vi "Image To From U32[].vi"(9 "U32[]":u32[](array[numeric]), 10 "Img In":T1) -> (1 "U32[] out":u32[](array[numeric]), 2 "Img":T1)   [LabVIEW 2021]
uses:
  <vilib>/picture/picture.llb/imagedata.ctl
  <vilib>/Utility/Data Type/NI_Data Type.lvlib
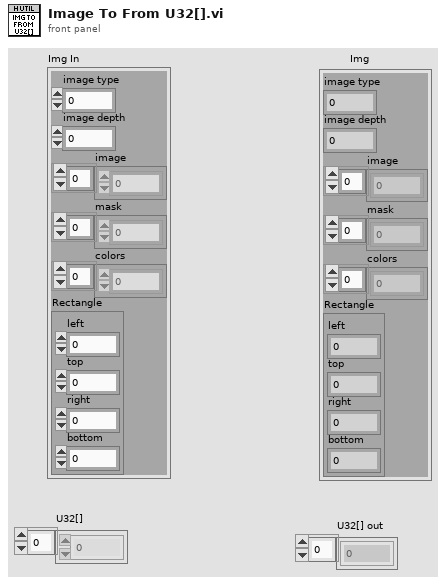
[diagram p1: front panel]
types:
  T1 = typedef "imagedata.ctl" = cluster{"image type":i32, "image depth":i32, "image":u8[], "mask":u8[], "colors":u32[], "Rectangle":cluster{"left":i16, "top":i16, "right":i16, "bottom":i16}}
  T2 = enum16{"Type", "Depth", "Sz & Image", "Sz & Mask", "Sz & Colors", "Rect"}
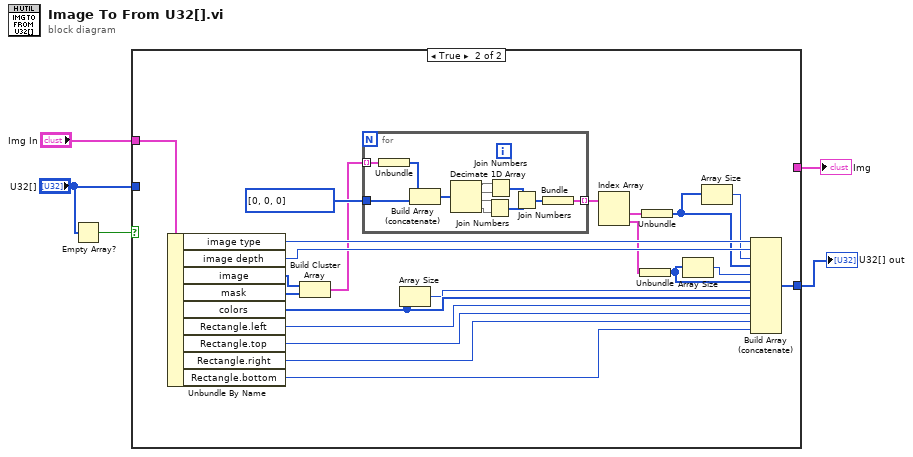
[diagram p0: block diagram]
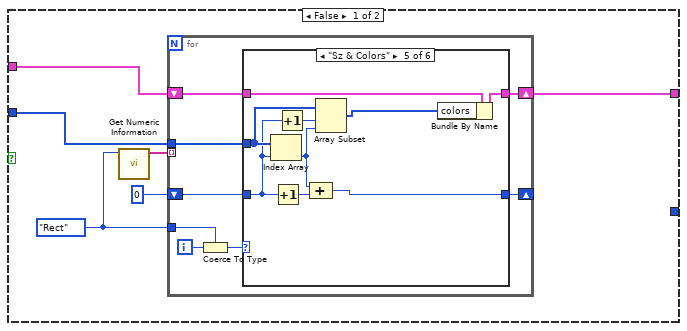
[diagram p2: hidden frame]
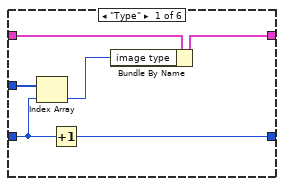
[diagram p3: hidden frame]
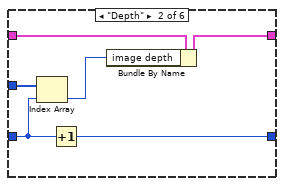
[diagram p4: hidden frame]
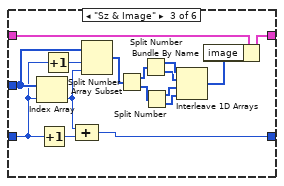
[diagram p5: hidden frame]
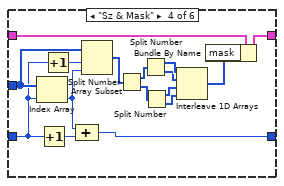
[diagram p6: hidden frame]
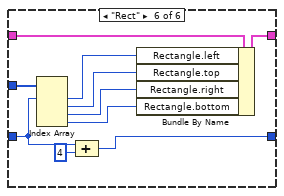
[diagram p7: hidden frame]
diagram:
  n1 = Empty Array?(array="U32[]") -> (empty?=w4:bool)
  n2 = case shown="True" w4 {
    tunnel: [w8 _] -> w5
    tunnel: "U32[]" -> [w7 _]
    tunnel: "Img In" -> [w6 w83]
    tunnel: [_ w84] -> w1
    frame False {
      w10 = T2."Rect"
      n3 = call <vilib>:"Get Numeric Information.vi"("variant"=w10) -> ("enum names"=w11:string[])  [unwired: 7 in, 3 out]
      n4 = for {
        shift-right: [w12] -> _
        shift-left: u32 0 -> [w14]
        tunnel: w7 -> [w16]
        tunnel: w11 -> [_] mode=indexing
        tunnel: w10 -> [w18]
        shift-right: [w13] -> w8
        shift-left: w6 -> [w15]
        i -> [w19]
        n5 = Coerce To Type(0:w19, 1:w18) -> (2:w17:T2)
        n6 = case shown="\"Sz & Colors\"" w17 {
          tunnel: w16 -> [w24 w30 w45 w61 w70 w80]
          tunnel: w15 -> [w25 w31 w47 w63 w72 w82]
          tunnel: w14 -> [w21 w27 w44 w60 w69 w78]
          tunnel: [w22 w28 w46 w62 w71 w81] -> w13
          tunnel: [w20 w26 w40 w56 w65 w79] -> w12
          frame "Type" {
            n7 = Index Array(array=w24, index=w21) -> (element=w23:u32)
            n8 = Increment(x=w21) -> (x+1=w20:u32)
            n9 = Bundle By Name(cluster=w25, "image type"=w23) -> (w22:T1)
          }
          frame "Depth" {
            n10 = Index Array(array=w30, index=w27) -> (element=w29:u32)
            n11 = Increment(x=w27) -> (x+1=w26:u32)
            n12 = Bundle By Name(cluster=w31, "image depth"=w29) -> (w28:T1)
          }
          frame "Sz & Image" {
            n13 = Index Array(array=w45, index=w44) -> (element=w41:u32)
            n14 = Increment(x=w44) -> (x+1=w42:u32)
            n15 = Increment(x=w44) -> (x+1=w43:u32)
            n16 = Compound Arithmetic op=ADD(w41, w42) -> (w40:u32)
            n17 = Array Subset(array=w45, index=w43, length=w41) -> (w39:u32[])
            n18 = Split Number(x=w39) -> (hi(x)=w38:u16[], lo(x)=w37:u16[])
            n19 = Split Number(x=w38) -> (hi(x)=w36:u8[], lo(x)=w35:u8[])
            n20 = Split Number(x=w37) -> (hi(x)=w34:u8[], lo(x)=w33:u8[])
            n21 = Interleave 1D Arrays(w36, w35, w34, w33) -> (w32:u8[])
            n22 = Bundle By Name(cluster=w47, "image"=w32) -> (w46:T1)
          }
          frame "Sz & Mask" {
            n23 = Index Array(array=w61, index=w60) -> (element=w57:u32)
            n24 = Increment(x=w60) -> (x+1=w58:u32)
            n25 = Increment(x=w60) -> (x+1=w59:u32)
            n26 = Compound Arithmetic op=ADD(w57, w58) -> (w56:u32)
            n27 = Array Subset(array=w61, index=w59, length=w57) -> (w55:u32[])
            n28 = Split Number(x=w55) -> (hi(x)=w54:u16[], lo(x)=w53:u16[])
            n29 = Split Number(x=w54) -> (hi(x)=w52:u8[], lo(x)=w51:u8[])
            n30 = Split Number(x=w53) -> (hi(x)=w50:u8[], lo(x)=w49:u8[])
            n31 = Interleave 1D Arrays(w52, w51, w50, w49) -> (w48:u8[])
            n32 = Bundle By Name(cluster=w63, "mask"=w48) -> (w62:T1)
          }
          frame "Sz & Colors" {
            n33 = Index Array(array=w70, index=w69) -> (element=w66:u32)
            n34 = Increment(x=w69) -> (x+1=w67:u32)
            n35 = Increment(x=w69) -> (x+1=w68:u32)
            n36 = Compound Arithmetic op=ADD(w66, w67) -> (w65:u32)
            n37 = Array Subset(array=w70, index=w68, length=w66) -> (w64:u32[])
            n38 = Bundle By Name(cluster=w72, "colors"=w64) -> (w71:T1)
          }
          frame "Rect" {
            n39 = Index Array(array=w80, index #1=w78) -> (element #1=w76:u32, element #2=w75:u32, element #3=w74:u32, element #4=w73:u32)  [unwired: 3 in]
            n40 = Compound Arithmetic op=ADD(w78, u32 4 ("value")) -> (w79:u32)
            n41 = Bundle By Name(cluster=w82, "Rectangle.left"=w76, "Rectangle.top"=w75, "Rectangle.right"=w74, "Rectangle.bottom"=w73) -> (w81:T1)
          }
        }
      }
    }
    frame True {
      n42 = Unbundle By Name(w83) -> ("image type"=w103:i32, "image depth"=w102:i32, "image"=w92:u8[], "mask"=w93:u8[], "colors"=w100:u32[], "Rectangle.left"=w101:i16, "Rectangle.top"=w98:i16, "Rectangle.right"=w97:i16, "Rectangle.bottom"=w96:i16)
      n43 = Build Cluster Array(w92, w93) -> (w91:cluster{"mask":u8[]}[])
      n44 = for {
        tunnel: u8[] [0, 0, 0] -> [w115]
        tunnel: [w104] -> w90 mode=indexing
        tunnel: w91 -> [w107] mode=indexing
        n45 = Unbundle(w107) -> ("mask"=w106:u8[])
        n46 = Build Array (concatenate)(w106, w115) -> (w114:u8[])
        n47 = Decimate 1D Array(w114) -> (w109:u8[], w108:u8[], w113:u8[], w112:u8[])
        n48 = Join Numbers(hi=w113, lo=w112) -> ((hi.lo)=w110:u16[])
        n49 = Join Numbers(hi=w109, lo=w108) -> ((hi.lo)=w111:u16[])
        n50 = Join Numbers(hi=w111, lo=w110) -> ((hi.lo)=w105:u32[])
        n51 = Bundle(w105) -> (w104:cluster{u32[]})  [unwired: 1 in]
      }
      n52 = Array Size(array=w100) -> (size(s)=w99:i32)
      n53 = Index Array(array=w90) -> (element #1=w89:cluster{u32[]}, element #2=w87:cluster{u32[]})  [unwired: 2 in]
      n54 = Unbundle(w87) -> (w86:u32[])
      n55 = Unbundle(w89) -> (w88:u32[])
      n56 = Array Size(array=w86) -> (size(s)=w85:i32)
      n57 = Array Size(array=w88) -> (size(s)=w94:i32)
      n58 = Build Array (concatenate)(w103, w102, w94, w88, w85, w86, w99, w100, w101, w98, w97, w96) -> (w84:u32[])
    }
  }
  "Img" <- w5
  "U32[] out" <- w1
